vi "setFactor.vi"(4 "Factor":u32, 5 "toFlash":bool, 6 "Error":bool, 7 "VISA resource name":refnum<visa-resource-name>="ASRL13::INSTR") -> (2 "Error":bool, 3 "dup VISA resource name":refnum<visa-resource-name>="ASRL13::INSTR")   [LabVIEW 2018]
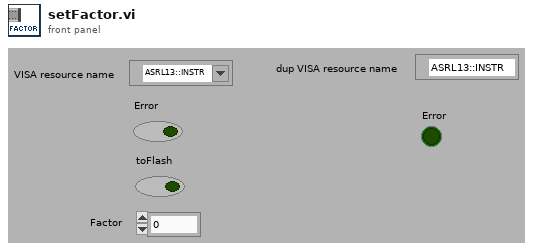
[diagram p1: front panel]
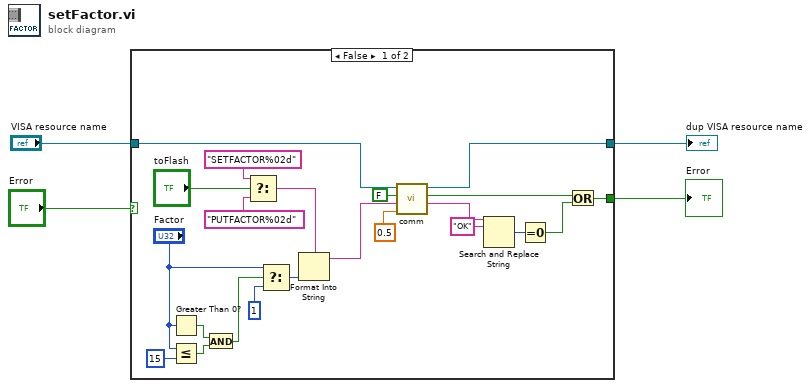
[diagram p0: block diagram]
diagram:
  n1 = case shown="False" "Error" {
    selector: "Error" -> [_ w28]
    tunnel: "VISA resource name" -> [w26 w27]
    tunnel: [w11 w28] -> w3
    tunnel: [w24 w27] -> w2
    frame False {
      n2 = Greater Than 0?(x="Factor") -> (x > 0?=w17:bool)
      n3 = Less Or Equal?(x="Factor", y=u32 15) -> (x <= y?=w16:bool)
      n4 = And(x=w17, y=w16) -> (x .and. y?=w15:bool)
      n5 = Select(t="SETFACTOR%02d" ("Substring"), s="toFlash", f="PUTFACTOR%02d" ("Substring")) -> (s? t:f=w5:string)
      n6 = Select(t="Factor", s=w15, f=u32 1) -> (s? t:f=w21:u32)
      n7 = Format Into String(format string=w5, w21) -> (resulting string=w25:string)  [unwired: 2 in, 1 out]
      n8 = call "comm.vi"("Timeout (s)"=0.5, "Command"=w25, "Error"=FALSE, "VISA resource name"=w26) -> ("Response"=w14:string, "Error"=w10:bool, "dup VISA resource name"=w24:refnum<visa-resource-name>)  [unwired: 2 in, 1 out]
      n9 = Search and Replace String(input string=w14, search string="OK") -> (number of replacements=w12:i32)  [unwired: 6 in, 3 out]
      n10 = Equal To 0?(x=w12) -> (x = 0?=w9:bool)
      n11 = Or(x=w10, y=w9) -> (x .or. y?=w11:bool)
    }
    frame True {
    }
  }
  "Error" <- w3
  "dup VISA resource name" <- w2
